vi "arrayadd.vi"(9 "b":dbl[](array[numeric]), 10 "a":dbl[](array[numeric])) -> (2 "c":dbl[](array[numeric]))   [LabVIEW 2012]
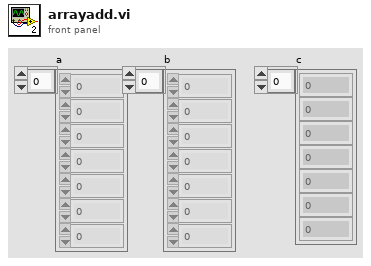
[diagram p1: front panel]
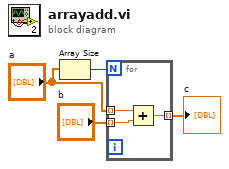
[diagram p0: block diagram]
diagram:
  n1 = Array Size(array="a") -> (size(s)=w4:i32)
  n2 = for {
    N: w4 -> [_]
    tunnel: "a" -> [w7] mode=indexing
    tunnel: "b" -> [w6] mode=indexing
    tunnel: [w5] -> w1 mode=indexing
    n3 = Add(x=w7, y=w6) -> (x+y=w5:dbl)
  }
  "c" <- w1
